vi "asAcq_dataWaitGet.vi"(0 "reference":refnum<class "OSA200.lvclass">, 2 "dataType":T1=enum."interferogram", 5 "error in (no error)":errorcluster, 7 "timeout (20000 ms)":i32=60000, 9 "error if timeout":bool=TRUE, 11 "ignore interfrgrm wLmt (OSA300)":bool=TRUE) -> (13 "timeOut":bool, 14 "duplicate reference":refnum<class "OSA200.lvclass">, 16 "dataType out":T1=enum."interferogram", 19 "error out":errorcluster)   [LabVIEW 2010, in "OSA200.lvclass"]
doc: "Waits for new data to be available and store retrieved data in a labview buffer, (see buffer_get.vi for data access)."
uses:
  OSA200.lvclass
  typeDef/acq_dataType.ctl
  OSA.lvclass
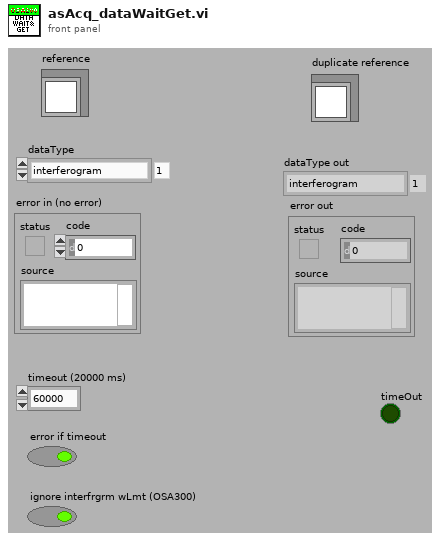
[diagram p1: front panel]
types:
  T1 = typedef "OSA.lvclass/acq_dataType.ctl" = enum16{"none", "interferogram", "spectrum"}
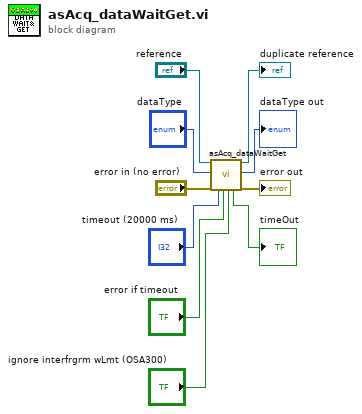
[diagram p0: block diagram]
diagram:
  n1 = call-parent "asAcq_dataWaitGet.vi"("reference"="reference", "dataType"="dataType", "error in (no error)"="error in (no error)", "timeout (20000 ms)"="timeout (20000 ms)", "error if timeout"="error if timeout", "ignore interfrgrm wLmt (OSA300)"="ignore interfrgrm wLmt (OSA300)") -> ("timeOut"=→"timeOut":bool, "duplicate reference"=→"duplicate reference":refnum<class "OSA200.lvclass">, "dataType out"=→"dataType out":T1, "error out"=→"error out":errorcluster)  [unwired: 10 in]
